vi "斯坦道XML解析.vi"(8 "error in (no error)":errorcluster, 9 "工作状态":u16, 10 "添加的路径":path, 11 "参数簇":cluster{"id":u16, "flowid":dbl, "range":dbl}={"id"=1, "flowid"=0.0, "range"=0.0}) -> (0 "error out":errorcluster, 2 "步骤名":string[][](array[string]), 3 "索引":string[](array[string]))   [LabVIEW 2016, in "斯坦道通用流路CODmn.lvlib"]
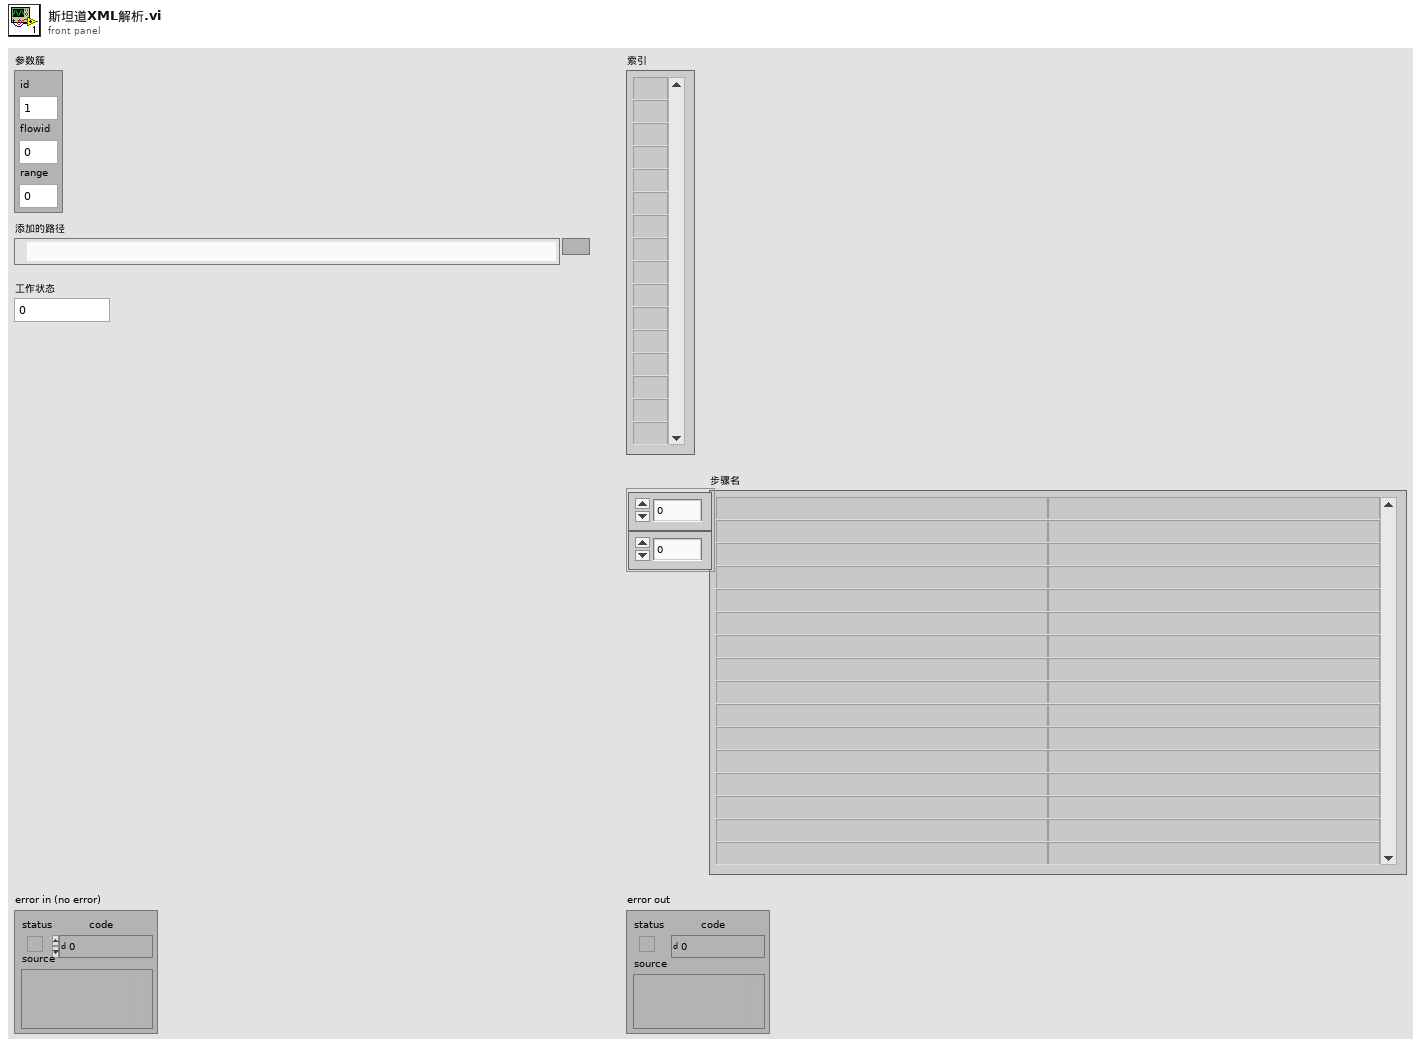
[diagram p1: front panel]
types:
  T1 = typedef "SingleStepTestV3.lvlib/SingleStepTestV3.lvclass/仪器版本.ctl" = enum16{"V3.1版", "V4版", "V3版", "V4.2版"}
  T2 = cluster{"port":i32, "dac":u8, "adc":u8, "time":u16, "步骤名":string}[]
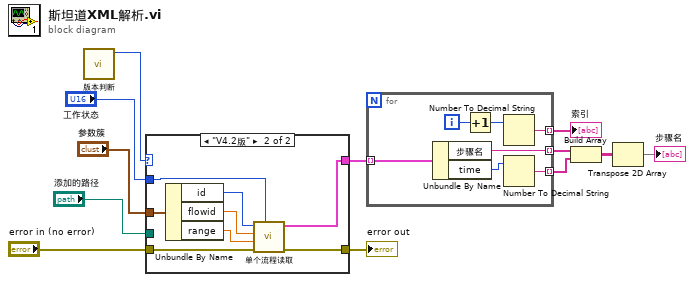
[diagram p0: block diagram]
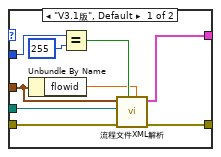
[diagram p2: hidden frame]
diagram:
  n1 = call "版本判断.vi"() -> ("仪器版本"=w1:T1)  [unwired: 11 in]
  n2 = case shown="\"V4.2版\"" w1 {
    tunnel: "添加的路径" -> [w21 _]
    tunnel: "参数簇" -> [w20 w28]
    tunnel: [w13 w22] -> w8
    tunnel: "error in (no error)" -> [w19 w23]
    tunnel: "工作状态" -> [w18 w24]
    tunnel: [w14 w29] -> w5
    frame "V3.1版", Default {
      n3 = Unbundle By Name(w20) -> ("flowid"=w15:dbl)
      n4 = Equal?(x=w18, y=u16 255) -> (x = y?=w16:bool)
      n5 = call "流程文件XML解析.vi"("简易流程Id"=w15, "是否是简易流程"=w16, "error in (no error)"=w19, "添加的路径"=w21, "参数簇"=w20) -> ("error out"=w13:errorcluster, "数组"=w14:T2)  [unwired: 5 in]
    }
    frame "V4.2版" {
      n6 = Unbundle By Name(w28) -> ("id"=w25:u16, "flowid"=w26:dbl, "range"=w27:dbl)
      n7 = call "单个流程读取.vi"("工作状态"=w24, "error in (no error)"=w23, "量程"=w27, "测量模式"=w26, "测量参数"=w25) -> ("error out"=w22:errorcluster, "数组 2"=w29:T2)  [unwired: 5 in]
    }
  }
  "error out" <- w8
  n8 = for {
    tunnel: w5 -> [w36] mode=indexing
    tunnel: [w34] -> w3 mode=indexing
    tunnel: [w33] -> w4 mode=indexing
    tunnel: [w30] -> w10 mode=indexing
    i -> [w32]
    n9 = Unbundle By Name(w36) -> ("步骤名"=w33:string, "time"=w35:u16)
    n10 = Increment(x=w32) -> (x+1=w31:i32)
    n11 = Number To Decimal String(number=w31) -> (decimal integer string=w30:string)  [unwired: 1 in]
    n12 = Number To Decimal String(number=w35) -> (decimal integer string=w34:string)  [unwired: 1 in]
  }
  "索引" <- w10
  n13 = Build Array(w4, w3) -> (w2:string[][])
  n14 = Transpose 2D Array(2D array=w2) -> (transposed array=→"步骤名":string[][])
